vi "testSetTempAndReadNamepathMap.vi"() -> ()   [LabVIEW 2017]
uses:
  Common/ObjectMap/LVPortObjectMapNamepathData.ctl
  Common/ObjectMap/LVPortObjectMapDataTypeEnum.ctl
  Common/ObjectMap/LVPortObjectMapContainerTypeEnum.ctl
panel:
  out "Updated":T1
  out "Matlab Param Data":T2[](array[typedef])
  in  "SomeVal":T1
  out "pID":string
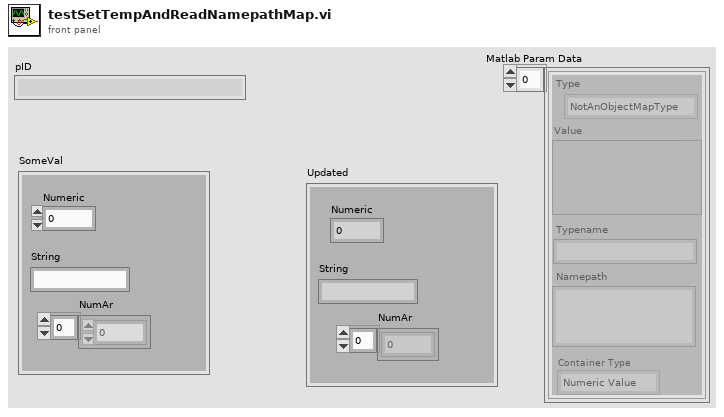
[diagram p1: front panel]
types:
  T1 = cluster{"Numeric":dbl, "String":string, "NumAr":dbl[]}
  T2 = typedef "LVPortObjectMapNamepathData.ctl" = cluster{"Type":T3, "Value":variant, "Namepath":string, "Typename":string, "Container Type":T4}
  T3 = typedef "LVPortObjectMapDataTypeEnum.ctl" = enum16{"NotAnObjectMapType", "Real", "Complex", "String", "Boolean"}
  T4 = typedef "LVPortObjectMapContainerTypeEnum.ctl" = enum16{"Numeric Value", "Numeric Array", "Waveform"}
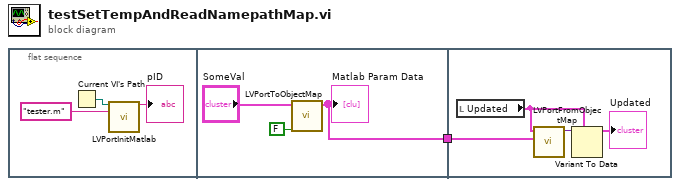
[diagram p0: block diagram]
diagram:
  n1 = flat-sequence {
    tunnel: [w6] -> w1
    tunnel: w1 -> [w11]
    frame #0 {
      n2 = Current VI's Path() -> (path=w4:path)
      n3 = call "LVPortInitMatlab.vi"("Working directory or VI Path"=w4, "Code file name"="tester.m") -> ("ID"=→"pID":string)  [unwired: 12 in, 1 out]
    }
    frame #1 {
      n4 = call "LVPortToObjectMap.vi"("Skip Parent Name (t)"=FALSE ("IgnoreContainerName"), "Value"="SomeVal") -> ("Object map"=w6:T2[])  [unwired: 9 in]
      "Matlab Param Data" <- w6
    }
    frame #2 {
      n5 = local read "Updated"() -> (w9:T1)
      n6 = call "LVPortFromObjectMap.vi"("Object Map"=w11, "Type (or value to update)"=w9) -> ("Value"=w10:variant)  [unwired: 9 in]
      n7 = Variant To Data(type=w9, Variant=w10) -> (data=→"Updated":T1)  [unwired: 1 in, 1 out]
    }
  }
